vi "Measurement Logic.vi"() -> ()   [LabVIEW 2021, in "IMD_Audio ADC.lvlib"]
uses:
  IMD_Audio ADC.lvlib
  shared/controls/Sync Commands.ctl
  shared/controls/Audio ADC Controls.lvlib
  shared/Audio ADC Shared.lvlib
  <vilib>/PDM Acquisition Toolkit/host/API/PDM Acquisition Toolkit.lvlib
  <resource>/objmgr/daqmx.rc
  <vilib>/PDM Acquisition Toolkit/host/API/Public/Read/Read PCM Input Waveform.vi
  <vilib>/PDM Acquisition Toolkit/host/API/Public/Start/Start PCM Input Task.vi
  <vilib>/DAQmx/create/channels.llb/DAQmx Create Channel (AO-Voltage-Basic).vi
  <vilib>/DAQmx/configure/timing.llb/DAQmx Timing (Sample Clock).vi
  <vilib>/PDM Acquisition Toolkit/host/API/Public/Clear/Clear PCM Input Task.vi
  Measurement Configuration.ctl
  Measurement Results.ctl
  <vilib>/Plug-In SDKs/Measurements/Measure Call Context/Measure Call Context.lvclass
panel:
  out "measurement results":T1
  in  "measurement configuration":T2={"Full scale range"=2.825, "Channel name"="", "Analog source resource name"="", "IMD standard"=enum."CCIF (11 kHz, 12 kHz, 1:1)", "Low frequency"=14000.0, "High frequency"=15000.0, "Amplitude ratio"=1.0, "Amplitude"=-1.0, "Protocol capture resource name"="", "Data line"=0, "Channel"=0, "Sample rate"=44100.0, "Measurement duration"=0.1, "Frame sync edge for Channel 0"=enum."Falling", "Channel count per frame"=2, "Channel length"=32, "Bit depth"=24, "Channel 0 offset"=1, "Endianness"=enum."MSB First", "Data Justification"=enum."Left Justified", "Frame length"=64, "Frame sync pulse width"=32, "Bit clock edge  sync"=enum."Falling"} {"High frequency" format="%#_pHz"; "Low frequency" format="%#_pHz"}
  out "error out":errorcluster
  out "measure call context out":refnum<class "Measure Call Context.lvclass">
  in  "measure call context in":refnum<class "Measure Call Context.lvclass">
  out "error out":errorcluster
  in  "error in":errorcluster
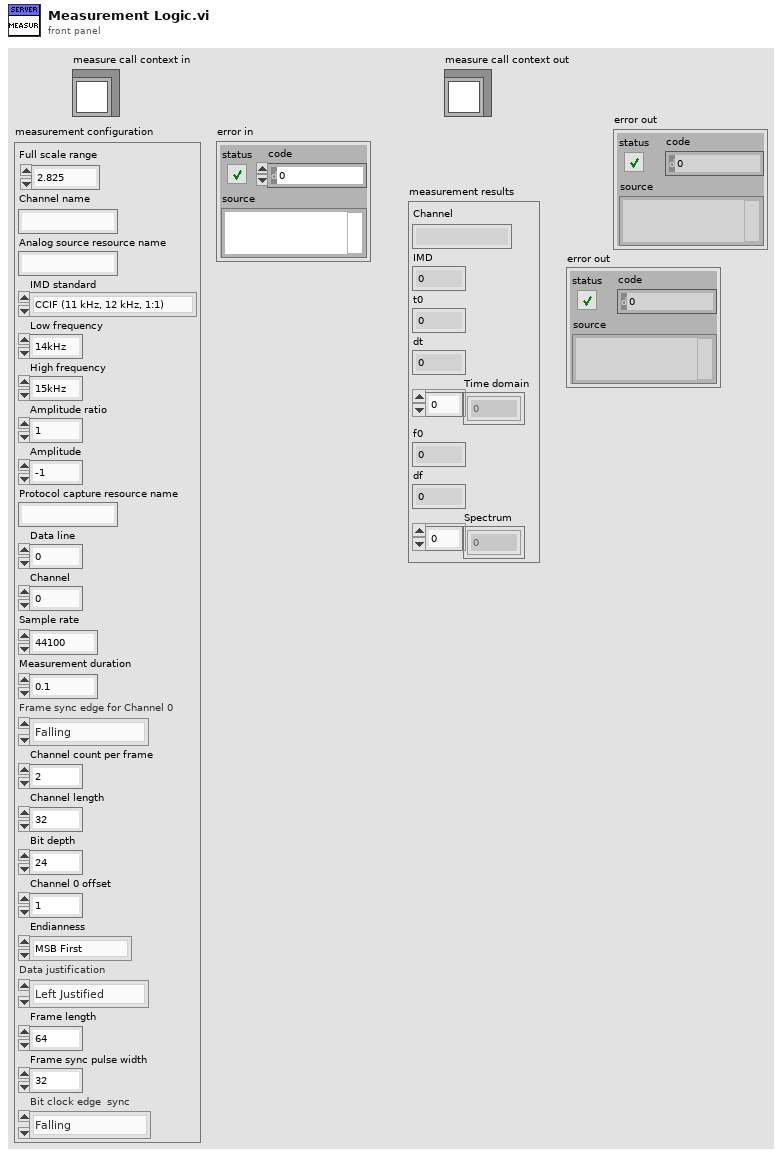
[diagram p1: front panel]
types:
  T1 = typedef "IMD_Audio ADC.lvlib/Measurement Results.ctl" = cluster{"Channel":string, "IMD":dbl, "t0":dbl, "dt":dbl, "Time domain":dbl[], "f0":dbl, "df":dbl, "Spectrum":dbl[]}
  T2 = typedef "IMD_Audio ADC.lvlib/Measurement Configuration.ctl" = cluster{"Full scale range":dbl, "Channel name":string, "Analog source resource name":string, "IMD standard":enum32{"SMPTE (60 Hz, 7000 Hz, 4:1)", "DIN (250 Hz, 8000 Hz, 4:1)", "CCIF (11 kHz, 12 kHz, 1:1)", "CCIF (19 kHz, 20 kHz, 1:1)", "Custom"}, "Low frequency":dbl, "High frequency":dbl, "Amplitude ratio":dbl, "Amplitude":dbl, "Protocol capture resource name":string, "Data line":u32, "Channel":u32, "Sample rate":dbl, "Measurement duration":dbl, "Frame sync edge for Channel 0":enum32{"Rising", "Falling"}, "Channel count per frame":u32, "Channel length":u32, "Bit depth":u32, "Channel 0 offset":u32, "Endianness":enum32{"MSB First", "LSB First"}, "Data Justification":enum32{"Left Justified", "Right Justified"}, "Frame length":u32, "Frame sync pulse width":u32, "Bit clock edge  sync":enum32{"Rising", "Falling"}}
  T3 = typedef "audio adc controls.lvlib/Sync Commands.ctl" = enum16{"NoAction", "GenerationStarted", "AcquisitionCompleted", "GenerationErrored"}
  T4 = typedef "Audio ADC Controls.lvlib/Protocol Settings Dual Channel.ctl" = cluster{"Protocol capture resource name":string, "Data line":u16, "Channel":string, "Clock rate":u32, "Number of words":i32, "Sensitivity":dbl, "Frame sync edge for channel 0":enum32{"Rising", "Falling"}, "Channel count per frame":u8, "Channel length":u16, "Bit depth":u8, "Channel 0 offset":u16, "Endianness":enum32{"MSB First", "LSB First"}, "Data justification":enum32{"Left Justified", "Right Justified"}, "Frame length":u16, "Frame sync pulse width":u16, "Bit clock edge sync":enum32{"Rising", "Falling"}}
  T5 = typedef "PDM Acquisition Class Library.lvlib/PCM Input Task.lvclass/DVR PCM Input Task.ctl" = refnum<data-value>
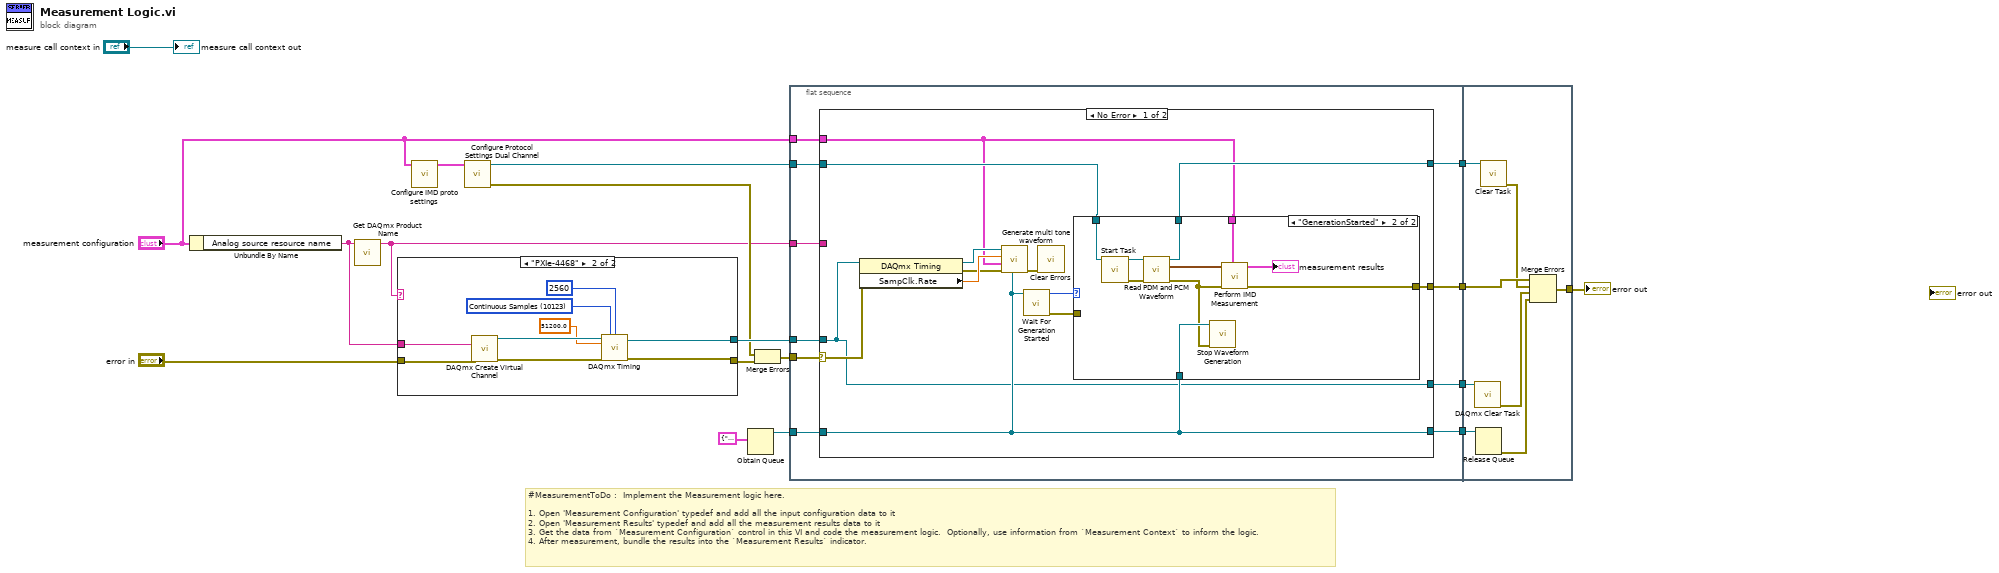
[diagram p0: block diagram]
diagram:
  # "#MeasurementToDo :  Implement the Measurement logic here.\n\n1. Open 'Measurement Configuration' typedef and add all the input configuration data to it\n2. Open 'Measurement Results' typedef and add all the measurement results data to it\n3. Get the data from `Measurement Configuration` control in this VI and code the measurement logic.  Optionally, use information from `Measurement Context` to inform the logic.\n4. After measurement, bundle the results into the `Measurement Results` indicator."
  n1 = Unbundle By Name("measurement configuration") -> ("Analog source resource name"=w14:string)
  n2 = call "Get DAQmx Product Name.vi"("DAQmx resource name"=w14) -> ("DAQmx product type"=w6:string)  [unwired: 10 in]
  n3 = case shown="\"PXIe-4468\"" w6 {
    tunnel: w14 -> [_ w28]
    tunnel: "error in" -> [w19 w22]
    tunnel: [w19 w20] -> w10
    tunnel: [_ w23] -> w12
    frame Default {
    }
    frame "PXIe-4468" {
      w25 = 10123 items=["Finite Samples"=10178, "Continuous Samples"=10123, "Hardware Timed Single Point"=12522] ("sample mode")
      n4 = call-poly <vilib>:"DAQmx Create Virtual Channel.vi"("physical channels"=w28, "error in"=w22) -> ("task out"=w27:refnum<k21>, "error out"=w21:errorcluster)  [unwired: 12 in]
      n5 = call-poly <vilib>:"DAQmx Timing.vi"("task/channels in"=w27, "sample mode"=w25, "samples per channel"=2560, "rate"=51200.0, "error in"=w21) -> ("task out"=w23:refnum<k21>, "error out"=w20:errorcluster)  [unwired: 9 in]
    }
  }
  n6 = call "Configure IMD proto settings.vi"("measurement configuration"="measurement configuration") -> ("Protocol settings"=w4:T4)  [unwired: 10 in]
  n7 = call "Configure Protocol Settings Dual Channel.vi"("Protocol settings"=w4) -> ("error out"=w9:errorcluster, "PCM input task out"=w11:T5)  [unwired: 9 in]
  n8 = Obtain Queue(element data type=cluster{"Status":T3, "Error":errorcluster} {"Status"=enum."NoAction", "Error"={"status"=FALSE, "code"=0, "source"=""}}) -> (queue out=w7:refnum<queue>)  [unwired: 4 in, 2 out]
  n9 = Merge Errors(w9, w10) -> (w8:errorcluster)
  n10 = flat-sequence {
    tunnel: w12 -> [w34]
    tunnel: w7 -> [w31]
    tunnel: w8 -> [w32]
    tunnel: w11 -> [w38]
    tunnel: "measurement configuration" -> [w37]
    tunnel: [w30] -> w17
    tunnel: [w35] -> w16
    tunnel: [w36] -> w15
    tunnel: w6 -> [w33]
    tunnel: [w29] -> w1
    tunnel: w17 -> [w75]
    tunnel: w16 -> [w74]
    tunnel: w15 -> [w73]
    tunnel: [w70] -> w3
    tunnel: w1 -> [w69]
    frame #0 {
      n11 = case shown="No Error" w32 {
        selector: w32 -> [w40 w66]
        tunnel: w38 -> [w51 w67]
        tunnel: w37 -> [w41 _]
        tunnel: w31 -> [w44 w65]
        tunnel: [w46 w66] -> w36
        tunnel: [w50 w67] -> w35
        tunnel: w34 -> [w39 w64]
        tunnel: w33 -> [_ _]
        tunnel: [w44 w65] -> w30
        tunnel: [w39 w64] -> w29
        frame No Error {
          n12 = property class="DAQmx Timing"(reference=w39, error in=w40) -> (reference out=w49:refnum<k21>, error out=w47:errorcluster, "SampClk.Rate"=w48:dbl)
          n13 = call "Generate multi tone waveform.vi"("hardware commands sync queue"=w44, "error in"=w47, "measurement configuration"=w41, "Sample Rate (Hz)"=w48, "task/channels in"=w49) -> ("error out"=w42:errorcluster)  [unwired: 5 in, 1 out]
          n14 = call "Wait For Generation Started.vi"("hardware commands sync queue"=w44) -> ("error out"=w43:errorcluster, "Status"=w45:T3)  [unwired: 9 in]
          n15 = call <vilib>:"Clear Errors.vi"("error in (no error)"=w42) -> ()  [unwired: 5 in, 2 out]
          n16 = case shown="\"GenerationStarted\"" w45 {
            tunnel: w51 -> [w52 w63]
            tunnel: [w52 w62] -> w50
            tunnel: w41 -> [_ w61]
            tunnel: [w53 w60] -> w46
            tunnel: w44 -> [_ w59]
            tunnel: w43 -> [w53 _]
            frame "NoAction", Default {
            }
            frame "GenerationStarted" {
              n17 = call-poly <vilib>:"Start Task.vi"("PCM input task in"=w63) -> ("error out"=w58:errorcluster, "PCM input task out"=w57:T5)  [unwired: 9 in]
              n18 = call-poly <vilib>:"Read PDM and PCM Waveform.vi"("error in"=w58, "PCM input task In"=w57) -> ("error out"=w54:errorcluster, "PCM waveforms"=w56:waveform(dbl)[], "PCM input task out"=w62:T5)  [unwired: 4 in, 3 out]
              n19 = call "Stop Waveform Generation.vi"("error in (no error)"=w54, "Hw sync command Q"=w59) -> ()  [unwired: 10 in]
              n20 = call "Perform IMD Measurement.vi"("measurement configuration"=w61, "error in"=w54, "PCM waveforms"=w56) -> ("error out"=w60:errorcluster, "measurement results"=→"measurement results":T1)  [unwired: 7 in]
            }
          }
        }
        frame Error {
        }
      }
    }
    frame #1 {
      n21 = call <vilib>:"DAQmx Clear Task.vi"("task in"=w69) -> ("error out"=w68:errorcluster)  [unwired: 14 in]
      n22 = Release Queue(queue=w75) -> (error out=w71:errorcluster)  [unwired: 2 in, 2 out]
      n23 = call-poly <vilib>:"Clear Task.vi"("PCM input task in"=w74) -> ("error out"=w72:errorcluster)  [unwired: 10 in]
      n24 = Merge Errors(w73, w72, w68, w71) -> (w70:errorcluster)
    }
  }
  "measure call context out" <- "measure call context in"
  "error out" <- w3
